vi "用户注册.vi"() -> ()   [LabVIEW 2020]
panel:
  in  "联系地址：":string
  in  "联系电话：":string
  in  "确认密码：":string
  in  "用户类型：":string(combo)="普通用户"
  in  "密      码：":string
  in  "用      户：":string
  in  "返回":bool
  in  "注册":bool
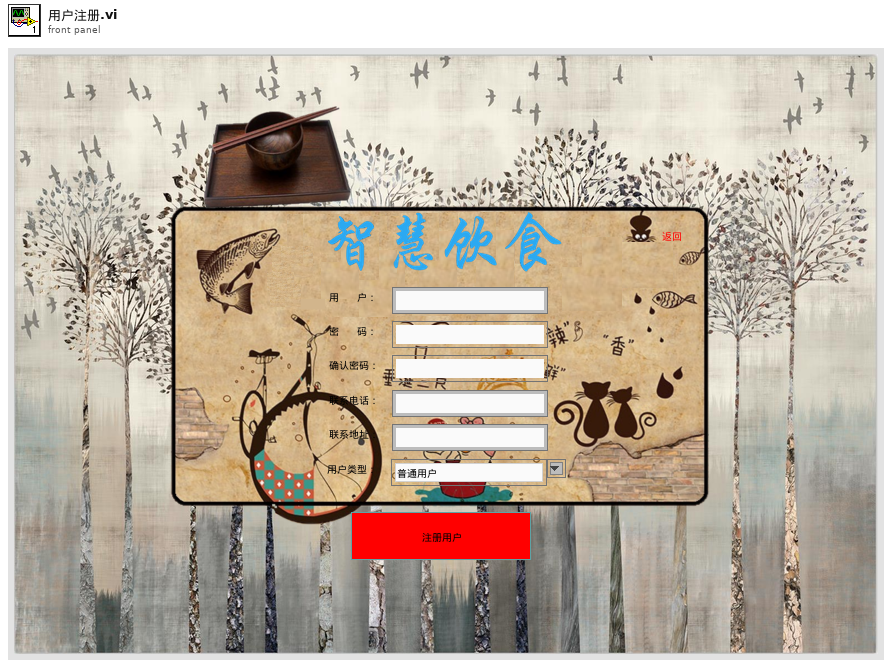
[diagram p1: front panel]
types:
  T1 = enum16{"write", "read", "read_key", "read_section"}
  T2 = typedef "Sound Output Task ID.ctl" = u32
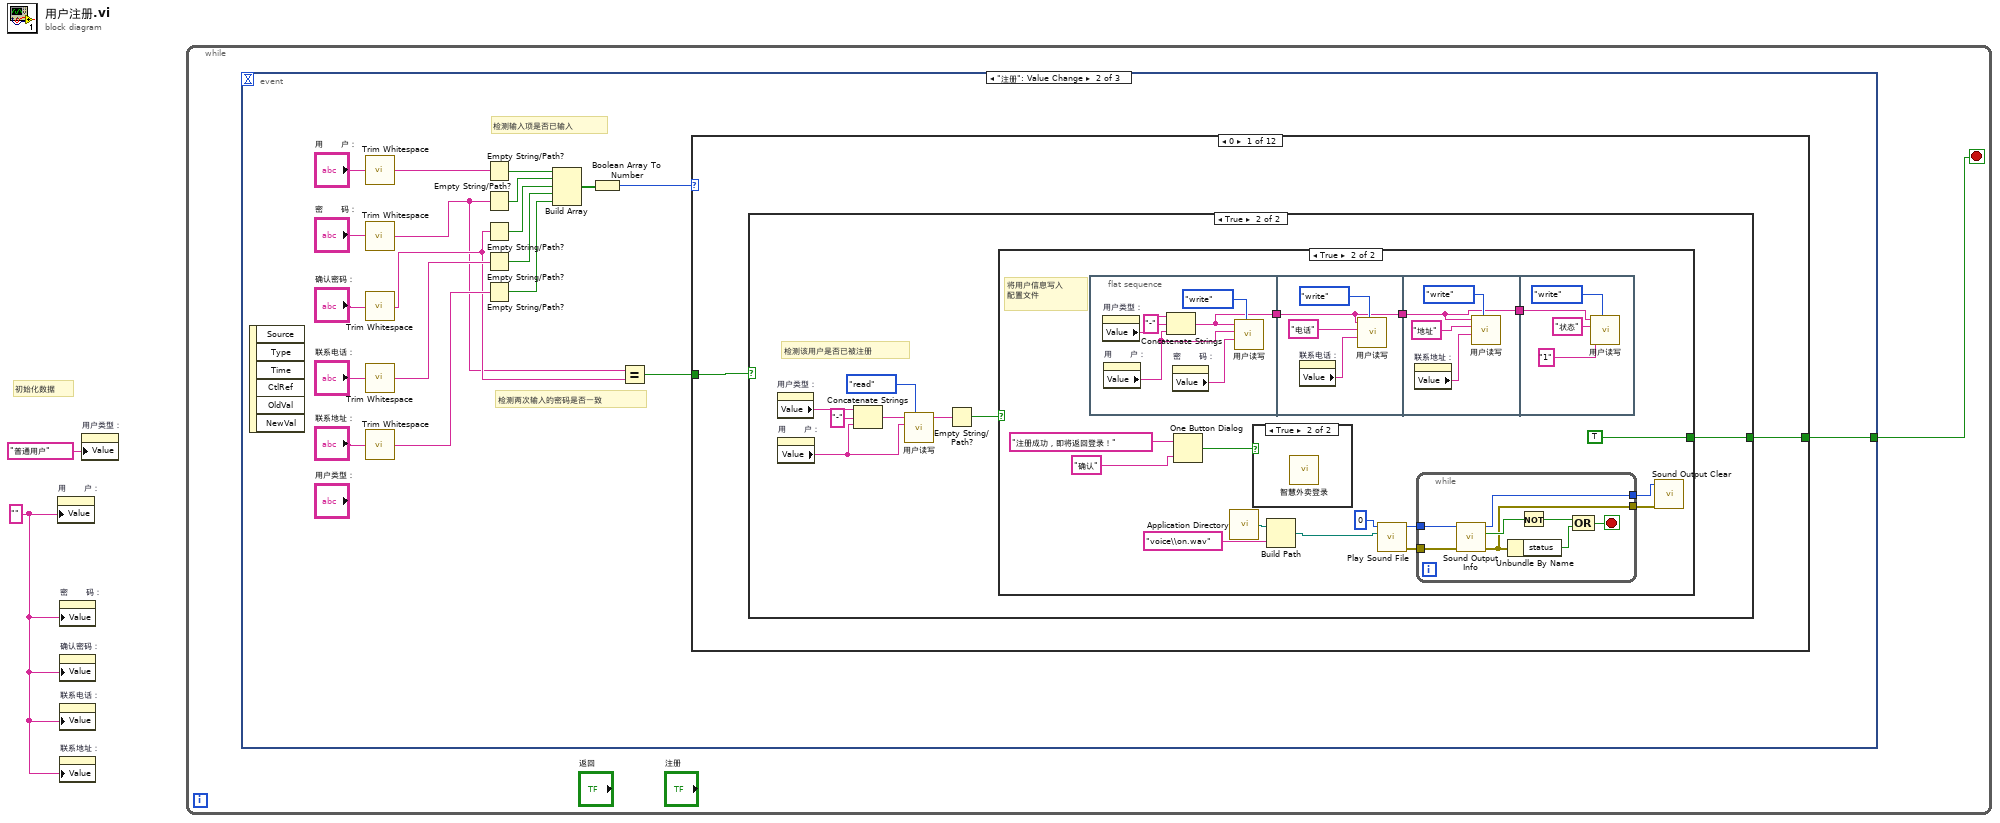
[diagram p0: block diagram]
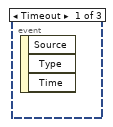
[diagram p2: hidden frame]
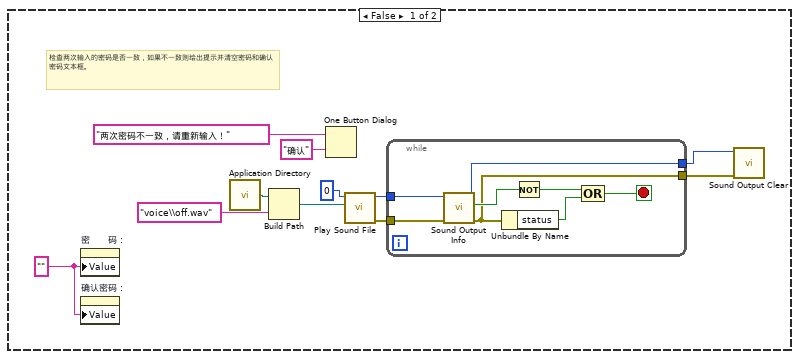
[diagram p3: hidden frame]
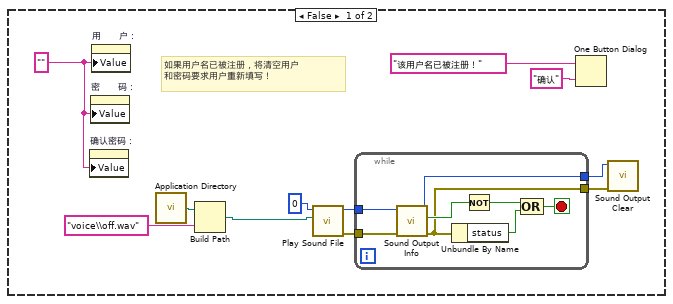
[diagram p4: hidden frame]
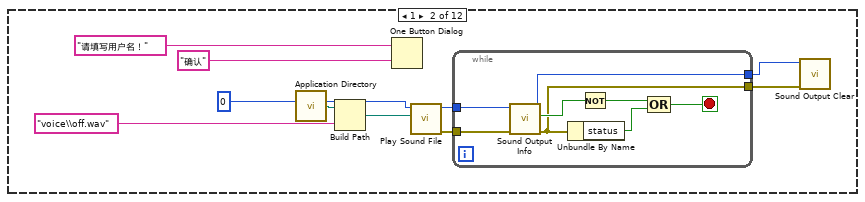
[diagram p6: hidden frame]
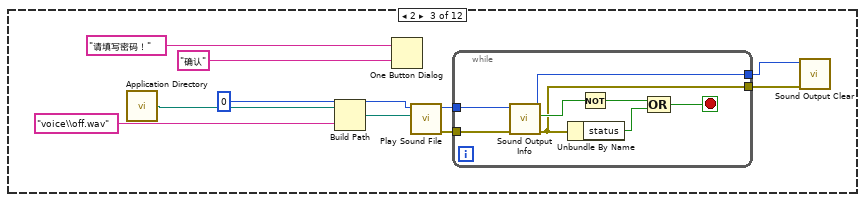
[diagram p7: hidden frame]
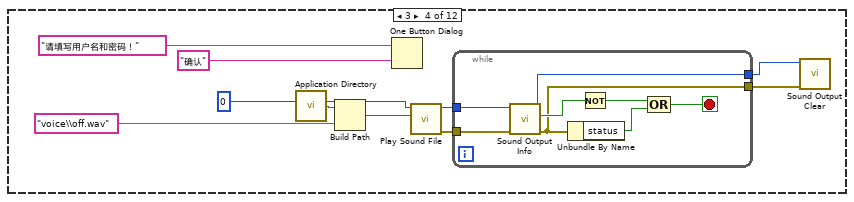
[diagram p8: hidden frame]
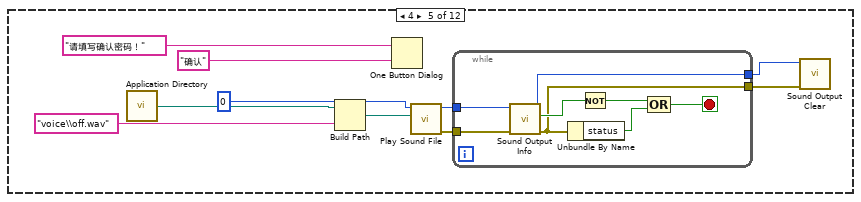
[diagram p9: hidden frame]
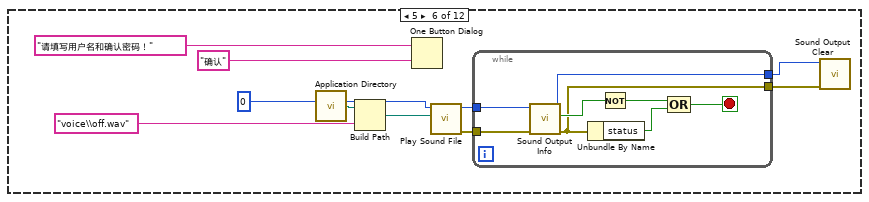
[diagram p10: hidden frame]
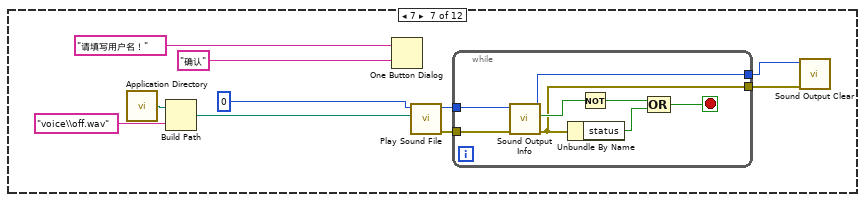
[diagram p11: hidden frame]
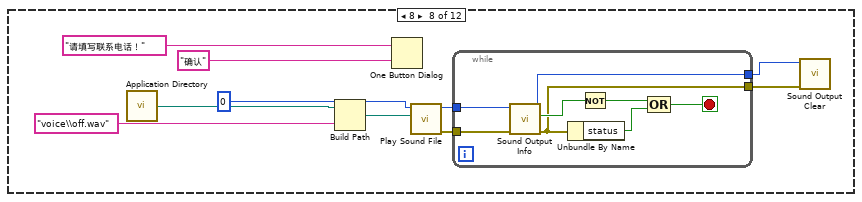
[diagram p12: hidden frame]
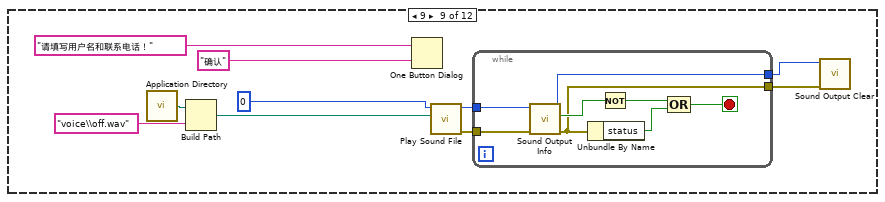
[diagram p13: hidden frame]
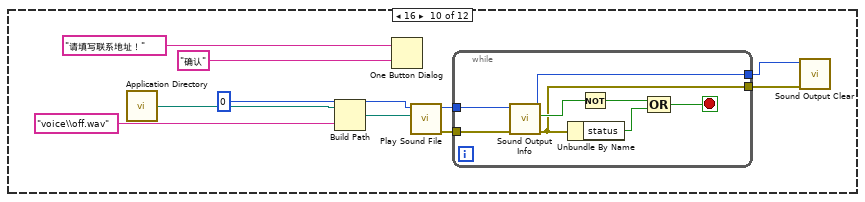
[diagram p14: hidden frame]
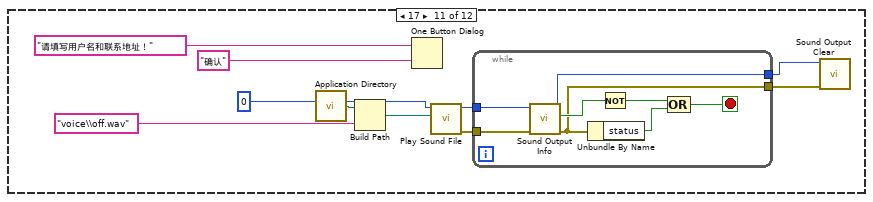
[diagram p15: hidden frame]
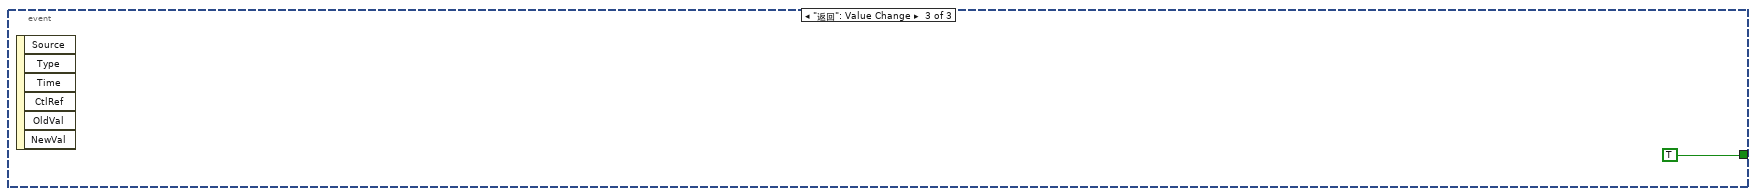
[diagram p17: hidden frame]
diagram:
  w1 = "" ("用户名：")
  # "初始化数据"
  n1 = property on="用      户：" class="Str"("Value"=w1) -> ()  [unwired: 2 in, 2 out]
  n2 = property on="密      码：" class="Str"("Value"=w1) -> ()  [unwired: 2 in, 2 out]
  n3 = property on="确认密码：" class="Str"("Value"=w1) -> ()  [unwired: 2 in, 2 out]
  n4 = property on="联系电话：" class="Str"("Value"=w1) -> ()  [unwired: 2 in, 2 out]
  n5 = property on="联系地址：" class="Str"("Value"=w1) -> ()  [unwired: 2 in, 2 out]
  n6 = property on="用户类型：" class="CmbBox"("Value"="普通用户" ("登录类型：")) -> ()  [unwired: 2 in, 2 out]
  n7 = while {
    stop <- w3 stop-if-true
    n8 = event shown="[1] \"注册\": Value Change" {
      selector: _ -> [_ _ _]
      dyn-events: _ -> [_ _ _]
      timeout: _ -> [_ _ _]
      tunnel: [_ w4 TRUE] -> w3
      event Timeout {
        n9 = event-data() -> ()  [unwired: 1 in, 3 out]
      }
      event "注册": Value Change {
        # "检测输入项是否已输入"
        # "检测两次输入的密码是否一致"
        n10 = event-data() -> ()  [unwired: 1 in, 6 out]
        n11 = call <vilib>:"Trim Whitespace.vi"("string"="用      户：") -> ("trimmed string"=w7:string)  [unwired: 1 in]
        n12 = call <vilib>:"Trim Whitespace.vi"("string"="密      码：") -> ("trimmed string"=w8:string)  [unwired: 1 in]
        n13 = call <vilib>:"Trim Whitespace.vi"("string"="确认密码：") -> ("trimmed string"=w9:string)  [unwired: 1 in]
        n14 = call <vilib>:"Trim Whitespace.vi"("string"="联系电话：") -> ("trimmed string"=w10:string)  [unwired: 1 in]
        n15 = call <vilib>:"Trim Whitespace.vi"("string"="联系地址：") -> ("trimmed string"=w11:string)  [unwired: 1 in]
        n16 = Empty String/Path?(string/path=w7) -> (empty?=w22:bool)
        n17 = Empty String/Path?(string/path=w8) -> (empty?=w21:bool)
        n18 = Empty String/Path?(string/path=w9) -> (empty?=w20:bool)
        n19 = Empty String/Path?(string/path=w10) -> (empty?=w19:bool)
        n20 = Empty String/Path?(string/path=w11) -> (empty?=w18:bool)
        n21 = Build Array(w22, w21, w20, w19, w18) -> (w17:bool[])
        n22 = Boolean Array To Number(Boolean array=w17) -> (number=w6:u32)
        n23 = Equal?(x=w8, y=w9) -> (x = y?=w5:bool)
        n24 = case shown="0" w6 {
          tunnel: w5 -> [w24 _ _ _ _ _ _ _ _ _ _ _]
          tunnel: [w23 _ _ _ _ _ _ _ _ _ _ _] -> w4
          frame 0 {
            n25 = case shown="True" w24 {
              tunnel: [_ w44] -> w23
              frame False {
                w25 = "" ("密      码：")
                # "检查两次输入的密码是否一致，如果不一致则给出提示并清空密码和确认密码文本框。"
                n26 = property on="密      码：" class="Str"("Value"=w25) -> ()  [unwired: 2 in, 2 out]
                n27 = property on="确认密码：" class="Str"("Value"=w25) -> ()  [unwired: 2 in, 2 out]
                n28 = call <vilib>:"Application Directory.vi"() -> ("Application Directory"=w35:path)
                n29 = Build Path(base path=w35, name or relative path="voice\\off.wav" ("名称或相对路径")) -> (appended path=w30:path)
                n30 = One Button Dialog(message="两次密码不一致，请重新输入！" ("消息"), button name ("OK")="确认" ("按钮名称（“确定”）")) -> ()  [unwired: 1 out]
                n31 = call <vilib>:"Play Sound File.vi"("path"=w30, "device ID"=u32 0) -> ("error out"=w34:errorcluster, "task ID"=w33:T2)  [unwired: 8 in]
                n32 = while {
                  tunnel: w34 -> [w43]
                  tunnel: w33 -> [w42]
                  tunnel: [w37] -> w32
                  tunnel: [w36] -> w31
                  stop <- w39 stop-if-true
                  n33 = call <vilib>:"Sound Output Info.vi"("error in (no error)"=w43, "task ID"=w42) -> ("error out"=w36:errorcluster, "is playing?"=w41:bool, "task ID out"=w37:T2)  [unwired: 6 in, 1 out]
                  n34 = Unbundle By Name(w36) -> ("status"=w38:bool)
                  n35 = Not(x=w41) -> (.not. x?=w40:bool)
                  n36 = Compound Arithmetic op=OR(w40, w38) -> (w39:bool)
                }
                n37 = call <vilib>:"Sound Output Clear.vi"("error in (no error)"=w31, "task ID"=w32) -> ()  [unwired: 9 in, 1 out]
              }
              frame True {
                # "检测该用户是否已被注册"
                n38 = property on="用户类型：" class="CmbBox"() -> ("Value"=w51:string)  [unwired: 2 in, 2 out]
                n39 = property on="用      户：" class="Str"() -> ("Value"=w47:string)  [unwired: 2 in, 2 out]
                n40 = Concatenate Strings(w51, "-" ("string"), w47) -> (w48:string)
                n41 = call "用户读写.vi"("Enum"=T1."read", "键"=w47, "字段"=w48) -> ("读取到的值"=w46:string)  [unwired: 6 in, 2 out]
                n42 = Empty String/Path?(string/path=w46) -> (empty?=w45:bool)
                n43 = case shown="True" w45 {
                  tunnel: [_ TRUE] -> w44
                  frame False {
                    w52 = "" ("用      户：")
                    # "如果用户名已被注册，将清空用户\n和密码要求用户重新填写！"
                    n44 = property on="确认密码：" class="Str"("Value"=w52) -> ()  [unwired: 2 in, 2 out]
                    n45 = property on="密      码：" class="Str"("Value"=w52) -> ()  [unwired: 2 in, 2 out]
                    n46 = property on="用      户：" class="Str"("Value"=w52) -> ()  [unwired: 2 in, 2 out]
                    n47 = call <vilib>:"Application Directory.vi"() -> ("Application Directory"=w57:path)
                    n48 = Build Path(base path=w57, name or relative path="voice\\off.wav" ("名称或相对路径")) -> (appended path=w62:path)
                    n49 = call <vilib>:"Play Sound File.vi"("path"=w62, "device ID"=u32 0) -> ("error out"=w58:errorcluster, "task ID"=w59:T2)  [unwired: 8 in]
                    n50 = while {
                      tunnel: w58 -> [w70]
                      tunnel: w59 -> [w69]
                      tunnel: [w64] -> w60
                      tunnel: [w63] -> w61
                      stop <- w66 stop-if-true
                      n51 = call <vilib>:"Sound Output Info.vi"("error in (no error)"=w70, "task ID"=w69) -> ("error out"=w63:errorcluster, "is playing?"=w68:bool, "task ID out"=w64:T2)  [unwired: 6 in, 1 out]
                      n52 = Unbundle By Name(w63) -> ("status"=w65:bool)
                      n53 = Not(x=w68) -> (.not. x?=w67:bool)
                      n54 = Compound Arithmetic op=OR(w67, w65) -> (w66:bool)
                    }
                    n55 = One Button Dialog(message="该用户名已被注册！" ("消息"), button name ("OK")="确认" ("按钮名称（“确定”）")) -> ()  [unwired: 1 out]
                    n56 = call <vilib>:"Sound Output Clear.vi"("error in (no error)"=w61, "task ID"=w60) -> ()  [unwired: 9 in, 1 out]
                  }
                  frame True {
                    # "将用户信息写入\n配置文件"
                    n57 = flat-sequence {
                      tunnel: [w86] -> w74
                      tunnel: w74 -> [w92]
                      tunnel: [w92] -> w73
                      tunnel: w73 -> [w96]
                      tunnel: [w96] -> w72
                      tunnel: w72 -> [w102]
                      frame #0 {
                        n58 = property on="用户类型：" class="CmbBox"() -> ("Value"=w91:string)  [unwired: 2 in, 2 out]
                        n59 = property on="用      户：" class="Str"() -> ("Value"=w89:string)  [unwired: 2 in, 2 out]
                        n60 = Concatenate Strings(w91, "-" ("string"), w89) -> (w86:string)
                        n61 = property on="密      码：" class="Str"() -> ("Value"=w88:string)  [unwired: 2 in, 2 out]
                        n62 = call "用户读写.vi"("Enum"=T1."write", "值"=w88, "键"=w89, "字段"=w86) -> ()  [unwired: 5 in, 3 out]
                      }
                      frame #1 {
                        n63 = property on="联系电话：" class="Str"() -> ("Value"=w93:string)  [unwired: 2 in, 2 out]
                        n64 = call "用户读写.vi"("Enum"=T1."write", "值"=w93, "键"="电话", "字段"=w92) -> ()  [unwired: 5 in, 3 out]
                      }
                      frame #2 {
                        n65 = property on="联系地址：" class="Str"() -> ("Value"=w97:string)  [unwired: 2 in, 2 out]
                        n66 = call "用户读写.vi"("Enum"=T1."write", "值"=w97, "键"="地址", "字段"=w96) -> ()  [unwired: 5 in, 3 out]
                      }
                      frame #3 {
                        n67 = call "用户读写.vi"("Enum"=T1."write", "值"="1", "键"="状态", "字段"=w102) -> ()  [unwired: 5 in, 3 out]
                      }
                    }
                    n68 = One Button Dialog(message="注册成功，即将返回登录！" ("消息"), button name ("OK")="确认" ("按钮名称（“确定”）")) -> (true=w83:bool)
                    n69 = call <vilib>:"Application Directory.vi"() -> ("Application Directory"=w75:path)
                    n70 = case shown="True" w83 {
                      frame False {
                      }
                      frame True {
                        n71 = call "智慧外卖登录.vi"() -> ()  [unwired: 12 in]
                      }
                    }
                    n72 = Build Path(base path=w75, name or relative path="voice\\on.wav" ("名称或相对路径")) -> (appended path=w82:path)
                    n73 = call <vilib>:"Play Sound File.vi"("path"=w82, "device ID"=u32 0) -> ("error out"=w78:errorcluster, "task ID"=w79:T2)  [unwired: 8 in]
                    n74 = while {
                      tunnel: w78 -> [w111]
                      tunnel: w79 -> [w110]
                      tunnel: [w105] -> w80
                      tunnel: [w104] -> w81
                      stop <- w107 stop-if-true
                      n75 = call <vilib>:"Sound Output Info.vi"("error in (no error)"=w111, "task ID"=w110) -> ("error out"=w104:errorcluster, "is playing?"=w109:bool, "task ID out"=w105:T2)  [unwired: 6 in, 1 out]
                      n76 = Unbundle By Name(w104) -> ("status"=w106:bool)
                      n77 = Not(x=w109) -> (.not. x?=w108:bool)
                      n78 = Compound Arithmetic op=OR(w108, w106) -> (w107:bool)
                    }
                    n79 = call <vilib>:"Sound Output Clear.vi"("error in (no error)"=w81, "task ID"=w80) -> ()  [unwired: 9 in, 1 out]
                  }
                }
              }
            }
          }
          frame 1 {
            n80 = call <vilib>:"Application Directory.vi"() -> ("Application Directory"=w121:path)
            n81 = Build Path(base path=w121, name or relative path="voice\\off.wav" ("名称或相对路径")) -> (appended path=w116:path)
            n82 = One Button Dialog(message="请填写用户名！" ("消息"), button name ("OK")="确认" ("按钮名称（“确定”）")) -> ()  [unwired: 1 out]
            n83 = call <vilib>:"Play Sound File.vi"("path"=w116, "device ID"=u32 0) -> ("error out"=w120:errorcluster, "task ID"=w119:T2)  [unwired: 8 in]
            n84 = while {
              tunnel: w120 -> [w129]
              tunnel: w119 -> [w128]
              tunnel: [w123] -> w118
              tunnel: [w122] -> w117
              stop <- w125 stop-if-true
              n85 = call <vilib>:"Sound Output Info.vi"("error in (no error)"=w129, "task ID"=w128) -> ("error out"=w122:errorcluster, "is playing?"=w127:bool, "task ID out"=w123:T2)  [unwired: 6 in, 1 out]
              n86 = Unbundle By Name(w122) -> ("status"=w124:bool)
              n87 = Not(x=w127) -> (.not. x?=w126:bool)
              n88 = Compound Arithmetic op=OR(w126, w124) -> (w125:bool)
            }
            n89 = call <vilib>:"Sound Output Clear.vi"("error in (no error)"=w117, "task ID"=w118) -> ()  [unwired: 9 in, 1 out]
          }
          frame 2 {
            n90 = call <vilib>:"Application Directory.vi"() -> ("Application Directory"=w139:path)
            n91 = Build Path(base path=w139, name or relative path="voice\\off.wav" ("名称或相对路径")) -> (appended path=w134:path)
            n92 = One Button Dialog(message="请填写密码！" ("消息"), button name ("OK")="确认" ("按钮名称（“确定”）")) -> ()  [unwired: 1 out]
            n93 = call <vilib>:"Play Sound File.vi"("path"=w134, "device ID"=u32 0) -> ("error out"=w138:errorcluster, "task ID"=w137:T2)  [unwired: 8 in]
            n94 = while {
              tunnel: w138 -> [w147]
              tunnel: w137 -> [w146]
              tunnel: [w141] -> w136
              tunnel: [w140] -> w135
              stop <- w143 stop-if-true
              n95 = call <vilib>:"Sound Output Info.vi"("error in (no error)"=w147, "task ID"=w146) -> ("error out"=w140:errorcluster, "is playing?"=w145:bool, "task ID out"=w141:T2)  [unwired: 6 in, 1 out]
              n96 = Unbundle By Name(w140) -> ("status"=w142:bool)
              n97 = Not(x=w145) -> (.not. x?=w144:bool)
              n98 = Compound Arithmetic op=OR(w144, w142) -> (w143:bool)
            }
            n99 = call <vilib>:"Sound Output Clear.vi"("error in (no error)"=w135, "task ID"=w136) -> ()  [unwired: 9 in, 1 out]
          }
          frame 3 {
            n100 = call <vilib>:"Application Directory.vi"() -> ("Application Directory"=w157:path)
            n101 = Build Path(base path=w157, name or relative path="voice\\off.wav" ("名称或相对路径")) -> (appended path=w152:path)
            n102 = One Button Dialog(message="请填写用户名和密码！" ("消息"), button name ("OK")="确认" ("按钮名称（“确定”）")) -> ()  [unwired: 1 out]
            n103 = call <vilib>:"Play Sound File.vi"("path"=w152, "device ID"=u32 0) -> ("error out"=w156:errorcluster, "task ID"=w155:T2)  [unwired: 8 in]
            n104 = while {
              tunnel: w156 -> [w165]
              tunnel: w155 -> [w164]
              tunnel: [w159] -> w154
              tunnel: [w158] -> w153
              stop <- w161 stop-if-true
              n105 = call <vilib>:"Sound Output Info.vi"("error in (no error)"=w165, "task ID"=w164) -> ("error out"=w158:errorcluster, "is playing?"=w163:bool, "task ID out"=w159:T2)  [unwired: 6 in, 1 out]
              n106 = Unbundle By Name(w158) -> ("status"=w160:bool)
              n107 = Not(x=w163) -> (.not. x?=w162:bool)
              n108 = Compound Arithmetic op=OR(w162, w160) -> (w161:bool)
            }
            n109 = call <vilib>:"Sound Output Clear.vi"("error in (no error)"=w153, "task ID"=w154) -> ()  [unwired: 9 in, 1 out]
          }
          frame 4 {
            n110 = call <vilib>:"Application Directory.vi"() -> ("Application Directory"=w175:path)
            n111 = Build Path(base path=w175, name or relative path="voice\\off.wav" ("名称或相对路径")) -> (appended path=w170:path)
            n112 = One Button Dialog(message="请填写确认密码！" ("消息"), button name ("OK")="确认" ("按钮名称（“确定”）")) -> ()  [unwired: 1 out]
            n113 = call <vilib>:"Play Sound File.vi"("path"=w170, "device ID"=u32 0) -> ("error out"=w174:errorcluster, "task ID"=w173:T2)  [unwired: 8 in]
            n114 = while {
              tunnel: w174 -> [w183]
              tunnel: w173 -> [w182]
              tunnel: [w177] -> w172
              tunnel: [w176] -> w171
              stop <- w179 stop-if-true
              n115 = call <vilib>:"Sound Output Info.vi"("error in (no error)"=w183, "task ID"=w182) -> ("error out"=w176:errorcluster, "is playing?"=w181:bool, "task ID out"=w177:T2)  [unwired: 6 in, 1 out]
              n116 = Unbundle By Name(w176) -> ("status"=w178:bool)
              n117 = Not(x=w181) -> (.not. x?=w180:bool)
              n118 = Compound Arithmetic op=OR(w180, w178) -> (w179:bool)
            }
            n119 = call <vilib>:"Sound Output Clear.vi"("error in (no error)"=w171, "task ID"=w172) -> ()  [unwired: 9 in, 1 out]
          }
          frame 5 {
            n120 = call <vilib>:"Application Directory.vi"() -> ("Application Directory"=w188:path)
            n121 = Build Path(base path=w188, name or relative path="voice\\off.wav" ("名称或相对路径")) -> (appended path=w193:path)
            n122 = One Button Dialog(message="请填写用户名和确认密码！" ("消息"), button name ("OK")="确认" ("按钮名称（“确定”）")) -> ()  [unwired: 1 out]
            n123 = call <vilib>:"Play Sound File.vi"("path"=w193, "device ID"=u32 0) -> ("error out"=w189:errorcluster, "task ID"=w190:T2)  [unwired: 8 in]
            n124 = while {
              tunnel: w189 -> [w201]
              tunnel: w190 -> [w200]
              tunnel: [w195] -> w191
              tunnel: [w194] -> w192
              stop <- w197 stop-if-true
              n125 = call <vilib>:"Sound Output Info.vi"("error in (no error)"=w201, "task ID"=w200) -> ("error out"=w194:errorcluster, "is playing?"=w199:bool, "task ID out"=w195:T2)  [unwired: 6 in, 1 out]
              n126 = Unbundle By Name(w194) -> ("status"=w196:bool)
              n127 = Not(x=w199) -> (.not. x?=w198:bool)
              n128 = Compound Arithmetic op=OR(w198, w196) -> (w197:bool)
            }
            n129 = call <vilib>:"Sound Output Clear.vi"("error in (no error)"=w192, "task ID"=w191) -> ()  [unwired: 9 in, 1 out]
          }
          frame 7 {
            n130 = call <vilib>:"Application Directory.vi"() -> ("Application Directory"=w211:path)
            n131 = Build Path(base path=w211, name or relative path="voice\\off.wav" ("名称或相对路径")) -> (appended path=w206:path)
            n132 = One Button Dialog(message="请填写用户名！" ("消息"), button name ("OK")="确认" ("按钮名称（“确定”）")) -> ()  [unwired: 1 out]
            n133 = call <vilib>:"Play Sound File.vi"("path"=w206, "device ID"=u32 0) -> ("error out"=w210:errorcluster, "task ID"=w209:T2)  [unwired: 8 in]
            n134 = while {
              tunnel: w210 -> [w219]
              tunnel: w209 -> [w218]
              tunnel: [w213] -> w208
              tunnel: [w212] -> w207
              stop <- w215 stop-if-true
              n135 = call <vilib>:"Sound Output Info.vi"("error in (no error)"=w219, "task ID"=w218) -> ("error out"=w212:errorcluster, "is playing?"=w217:bool, "task ID out"=w213:T2)  [unwired: 6 in, 1 out]
              n136 = Unbundle By Name(w212) -> ("status"=w214:bool)
              n137 = Not(x=w217) -> (.not. x?=w216:bool)
              n138 = Compound Arithmetic op=OR(w216, w214) -> (w215:bool)
            }
            n139 = call <vilib>:"Sound Output Clear.vi"("error in (no error)"=w207, "task ID"=w208) -> ()  [unwired: 9 in, 1 out]
          }
          frame 8 {
            n140 = call <vilib>:"Application Directory.vi"() -> ("Application Directory"=w224:path)
            n141 = Build Path(base path=w224, name or relative path="voice\\off.wav" ("名称或相对路径")) -> (appended path=w229:path)
            n142 = One Button Dialog(message="请填写联系电话！" ("消息"), button name ("OK")="确认" ("按钮名称（“确定”）")) -> ()  [unwired: 1 out]
            n143 = call <vilib>:"Play Sound File.vi"("path"=w229, "device ID"=u32 0) -> ("error out"=w225:errorcluster, "task ID"=w226:T2)  [unwired: 8 in]
            n144 = while {
              tunnel: w225 -> [w237]
              tunnel: w226 -> [w236]
              tunnel: [w231] -> w227
              tunnel: [w230] -> w228
              stop <- w233 stop-if-true
              n145 = call <vilib>:"Sound Output Info.vi"("error in (no error)"=w237, "task ID"=w236) -> ("error out"=w230:errorcluster, "is playing?"=w235:bool, "task ID out"=w231:T2)  [unwired: 6 in, 1 out]
              n146 = Unbundle By Name(w230) -> ("status"=w232:bool)
              n147 = Not(x=w235) -> (.not. x?=w234:bool)
              n148 = Compound Arithmetic op=OR(w234, w232) -> (w233:bool)
            }
            n149 = call <vilib>:"Sound Output Clear.vi"("error in (no error)"=w228, "task ID"=w227) -> ()  [unwired: 9 in, 1 out]
          }
          frame 9 {
            n150 = call <vilib>:"Application Directory.vi"() -> ("Application Directory"=w247:path)
            n151 = Build Path(base path=w247, name or relative path="voice\\off.wav" ("名称或相对路径")) -> (appended path=w242:path)
            n152 = One Button Dialog(message="请填写用户名和联系电话！" ("消息"), button name ("OK")="确认" ("按钮名称（“确定”）")) -> ()  [unwired: 1 out]
            n153 = call <vilib>:"Play Sound File.vi"("path"=w242, "device ID"=u32 0) -> ("error out"=w246:errorcluster, "task ID"=w245:T2)  [unwired: 8 in]
            n154 = while {
              tunnel: w246 -> [w255]
              tunnel: w245 -> [w254]
              tunnel: [w249] -> w244
              tunnel: [w248] -> w243
              stop <- w251 stop-if-true
              n155 = call <vilib>:"Sound Output Info.vi"("error in (no error)"=w255, "task ID"=w254) -> ("error out"=w248:errorcluster, "is playing?"=w253:bool, "task ID out"=w249:T2)  [unwired: 6 in, 1 out]
              n156 = Unbundle By Name(w248) -> ("status"=w250:bool)
              n157 = Not(x=w253) -> (.not. x?=w252:bool)
              n158 = Compound Arithmetic op=OR(w252, w250) -> (w251:bool)
            }
            n159 = call <vilib>:"Sound Output Clear.vi"("error in (no error)"=w243, "task ID"=w244) -> ()  [unwired: 9 in, 1 out]
          }
          frame 16 {
            n160 = call <vilib>:"Application Directory.vi"() -> ("Application Directory"=w265:path)
            n161 = Build Path(base path=w265, name or relative path="voice\\off.wav" ("名称或相对路径")) -> (appended path=w260:path)
            n162 = One Button Dialog(message="请填写联系地址！" ("消息"), button name ("OK")="确认" ("按钮名称（“确定”）")) -> ()  [unwired: 1 out]
            n163 = call <vilib>:"Play Sound File.vi"("path"=w260, "device ID"=u32 0) -> ("error out"=w264:errorcluster, "task ID"=w263:T2)  [unwired: 8 in]
            n164 = while {
              tunnel: w264 -> [w273]
              tunnel: w263 -> [w272]
              tunnel: [w267] -> w262
              tunnel: [w266] -> w261
              stop <- w269 stop-if-true
              n165 = call <vilib>:"Sound Output Info.vi"("error in (no error)"=w273, "task ID"=w272) -> ("error out"=w266:errorcluster, "is playing?"=w271:bool, "task ID out"=w267:T2)  [unwired: 6 in, 1 out]
              n166 = Unbundle By Name(w266) -> ("status"=w268:bool)
              n167 = Not(x=w271) -> (.not. x?=w270:bool)
              n168 = Compound Arithmetic op=OR(w270, w268) -> (w269:bool)
            }
            n169 = call <vilib>:"Sound Output Clear.vi"("error in (no error)"=w261, "task ID"=w262) -> ()  [unwired: 9 in, 1 out]
          }
          frame 17 {
            n170 = call <vilib>:"Application Directory.vi"() -> ("Application Directory"=w283:path)
            n171 = Build Path(base path=w283, name or relative path="voice\\off.wav" ("名称或相对路径")) -> (appended path=w278:path)
            n172 = One Button Dialog(message="请填写用户名和联系地址！" ("消息"), button name ("OK")="确认" ("按钮名称（“确定”）")) -> ()  [unwired: 1 out]
            n173 = call <vilib>:"Play Sound File.vi"("path"=w278, "device ID"=u32 0) -> ("error out"=w282:errorcluster, "task ID"=w281:T2)  [unwired: 8 in]
            n174 = while {
              tunnel: w282 -> [w291]
              tunnel: w281 -> [w290]
              tunnel: [w285] -> w280
              tunnel: [w284] -> w279
              stop <- w287 stop-if-true
              n175 = call <vilib>:"Sound Output Info.vi"("error in (no error)"=w291, "task ID"=w290) -> ("error out"=w284:errorcluster, "is playing?"=w289:bool, "task ID out"=w285:T2)  [unwired: 6 in, 1 out]
              n176 = Unbundle By Name(w284) -> ("status"=w286:bool)
              n177 = Not(x=w289) -> (.not. x?=w288:bool)
              n178 = Compound Arithmetic op=OR(w288, w286) -> (w287:bool)
            }
            n179 = call <vilib>:"Sound Output Clear.vi"("error in (no error)"=w279, "task ID"=w280) -> ()  [unwired: 9 in, 1 out]
          }
          frame 100, Default {
          }
        }
      }
      event "返回": Value Change {
        n180 = event-data() -> ()  [unwired: 1 in, 6 out]
      }
    }
  }
